vi "notifier with timeout MINI.vi"(8 "error constant":errorcluster, 9 "milliseconds to wait":u32=500, 11 "message":string="Success!") -> (0 "error out":errorcluster, 2 "cancel select":bool)   [LabVIEW 2015]
doc: "This is an example that shows how to have a message box pop up and exit with out having to press OK."
uses:
  user32.dll
panel:
  # "Overview: This is an example that shows how to have a message box pop up and exit with out having to press OK.\nRequirements: LabVIEW 2012 (or compatible)\nInstructions:\n1. Run the VI.\n2. When the window pop up, do nothing and the window will exit after several seconds."
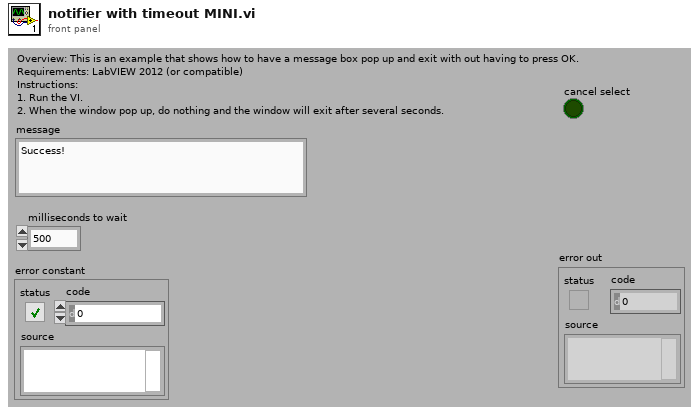
[diagram p1: front panel]
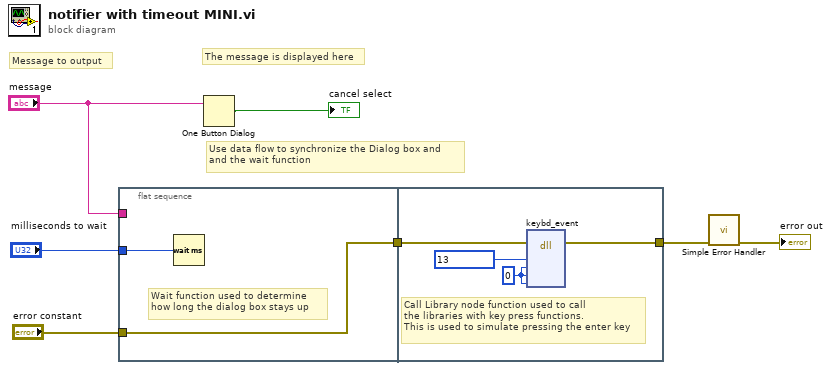
[diagram p0: block diagram]
diagram:
  # "The message is displayed here"
  # "Use data flow to synchronize the Dialog box and\nand the wait function"
  # "Message to output"
  n1 = flat-sequence {
    tunnel: "message" -> [_]
    tunnel: [w9] -> w4
    tunnel: "error constant" -> [w9]
    tunnel: "milliseconds to wait" -> [w8]
    tunnel: w4 -> [w10]
    tunnel: [w11] -> w6
    frame #0 {
      # "Wait function used to determine \nhow long the dialog box stays up"
      n2 = Wait (ms)(milliseconds to wait=w8) -> ()  [unwired: 1 out]
    }
    frame #1 {
      w12 = u8 0 ("bScan")
      # "Call Library node function used to call \nthe libraries with key press functions. \nThis is used to simulate pressing the enter key"
      n3 = dll-call lib="user32.dll" fn="keybd_event"(error in=w10, "bVk"=u8 13 ("Virtual Key"), "bScan"=w12, "dwFlags"=w12, "dwExtraInfo"=w12) -> (error out=w11:errorcluster)  [unwired: 7 in, 1 out]
    }
  }
  n4 = One Button Dialog(message="message") -> (true=→"cancel select":bool)  [unwired: 1 in]
  n5 = call <vilib>:"Simple Error Handler.vi"("error in (no error)"=w6) -> ("error out"=→"error out":errorcluster)  [unwired: 4 in, 4 out]
